vi "Disconnect.vi"(8 "error in (no error)":errorcluster, 11 "F4T in":refnum<class "F4T.lvclass">) -> (0 "error out":errorcluster, 3 "F4T out":refnum<class "F4T.lvclass">)   [LabVIEW 2018, in "F4T.lvlib" / "F4T.lvclass"]
uses:
  F4T.lvclass
  F4T.lvclass/F4T.ctl
  C:/Program Files/National Instruments/LabVIEW 2018/instr.lib/Watlow Std Bus/Public/Watbus.dll
  Program Files/National Instruments/LabVIEW 2018/instr.lib/Watlow Std Bus/Public/Watbus.dll
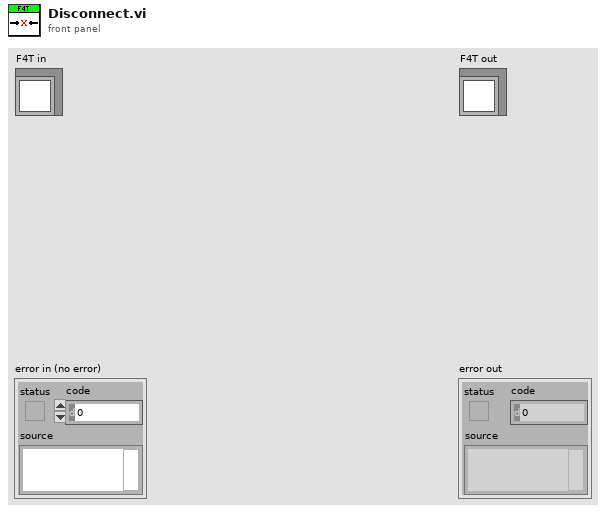
[diagram p1: front panel]
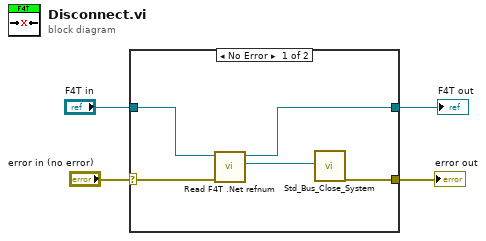
[diagram p0: block diagram]
diagram:
  n1 = case shown="No Error" "error in (no error)" {
    selector: "error in (no error)" -> [w8 w11]
    tunnel: [w9 w11] -> w3
    tunnel: "F4T in" -> [w6 w10]
    tunnel: [w5 w10] -> w1
    frame No Error {
      n2 = call "Read F4T .Net refnum.vi"("error in (no error)"=w8, "F4T in"=w6) -> ("F4T .Net refnum"=w7:refnum<k24>, "F4T out"=w5:refnum<class "F4T.lvclass">)  [unwired: 7 in, 1 out]
      n3 = call <instrlib>:"Std_Bus_Close_System.vi"("ILabVIEW In"=w7) -> ("error out"=w9:errorcluster)  [unwired: 18 in]
    }
    frame Error {
    }
  }
  "error out" <- w3
  "F4T out" <- w1
